vi "BRig_RT__Case_Exp__State_Cue.vi"(0 "input_dataCurrent":u16[](array[numeric]), 1 "input_dataTrial":u16[][](array[numeric]), 5 "input_arrTrig":bool[](array[boolean]), 6 "input_state":T1, 8 "I_lick":bool) -> (7 "output_l2_laserOn":bool, 9 "output_l2_laserEvent":bool, 10 "output_SelectionState":bool, 11 "output_l1_laserOn":bool, 12 "output_state":T1, 13 "output_l1_laserEvent":bool, 14 "output_dataCurrent":u16[](array[numeric]), 15 "output_dataTrial":u16[][](array[numeric]), 17 "output_CueLed":bool, 18 "output_Audio_L":bool, 19 "output_Audio_R":bool)   [LabVIEW 2014]
uses:
  myRIO_BRig_RT__Case_Exp_stateList.ctl
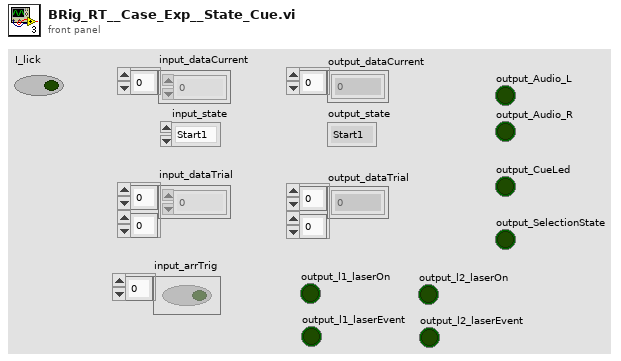
[diagram p1: front panel]
types:
  T1 = typedef "myRIO_BRig_RT__Case_Exp_stateList.ctl" = enum16{"Start1", "Start2", "Start3", "saveSettings1", "saveSettings2", "saveSettings3", "saveSettings4", "saveSettings_LC_ENL_l1", "saveSettings_LC_ENL_l2", "saveSettings_LC_Cue_l1", "saveSettings_LC_Cue_l2", "saveSettings6_LC_l1_Other", "SaveSettings6_LC_l2_Other", "setSettings_Audio", "setSettings_Laser", "initBlock_pre", "initBlock", "initBlock2", "initBlock_post", "initTrial_pre", "initTrial", "initTrial2", "initTrial3", "initTrial4", "initTrial_LC_ENL1", "initTrial_LC_Cue1", "initTrial_LC_Cue1_2", "initTrial_LC_Sel", "initTrial_post", "ENL1_pre", "ENL1", "ENL1_post", "ENL1Penalty_pre", "ENL1Penalty", "ENL2_pre", "ENL2", "ENL2Penalty_pre", "ENL2Penalty", "Cue1_pre", "Cue1", "Cue1_post", "Cue1Penalty_pre", "Cue1Penalty", "Cue2_pre", "Cue2", "Cue2Penalty_pre", "Cue2Penalty", "Selection_pre", "Selection", "Select_post", "SelectReward_pre", "SelectReward", "SelectRewardPost_pre", "SelectRewardPost", "SelectWrong_pre", "SelectWrong", "SelectWrong_post", "SelectTimeout_pre", "SelectTimeout", "SelectTimeout_post", "endTrial_pre", "endTrial1", "endTrial2", "endTrial3", "endTrial_post", "endBlock_pre", "endBlock", "endBlock_post", "endExp", "commConnect", "commUpload_pre", "commUpload_dataBlock", "commUpload_dataCurrent", "commUpload_dataExp", "commUpload_dataLC", "commUpload_dataTrial", "commUpload_post", "saveData_pre", "saveData_dataBlock", "saveData_dataCurrent", "saveData_dataExp", "saveData_dataLC", "saveData_dataTrial", "saveData_post", "empty_endBlock1", "empty_endBlock2", "empty_endTrial1", "empty_endTrial2", "empty_endTrial3", "empty_endTrial4", "empty_endTrial5", "dummyState", "dummyState_endBlock", "FreeReward_pre", "FreeReward", "FreeRewardPost_pre", "FreeRewardPost"}
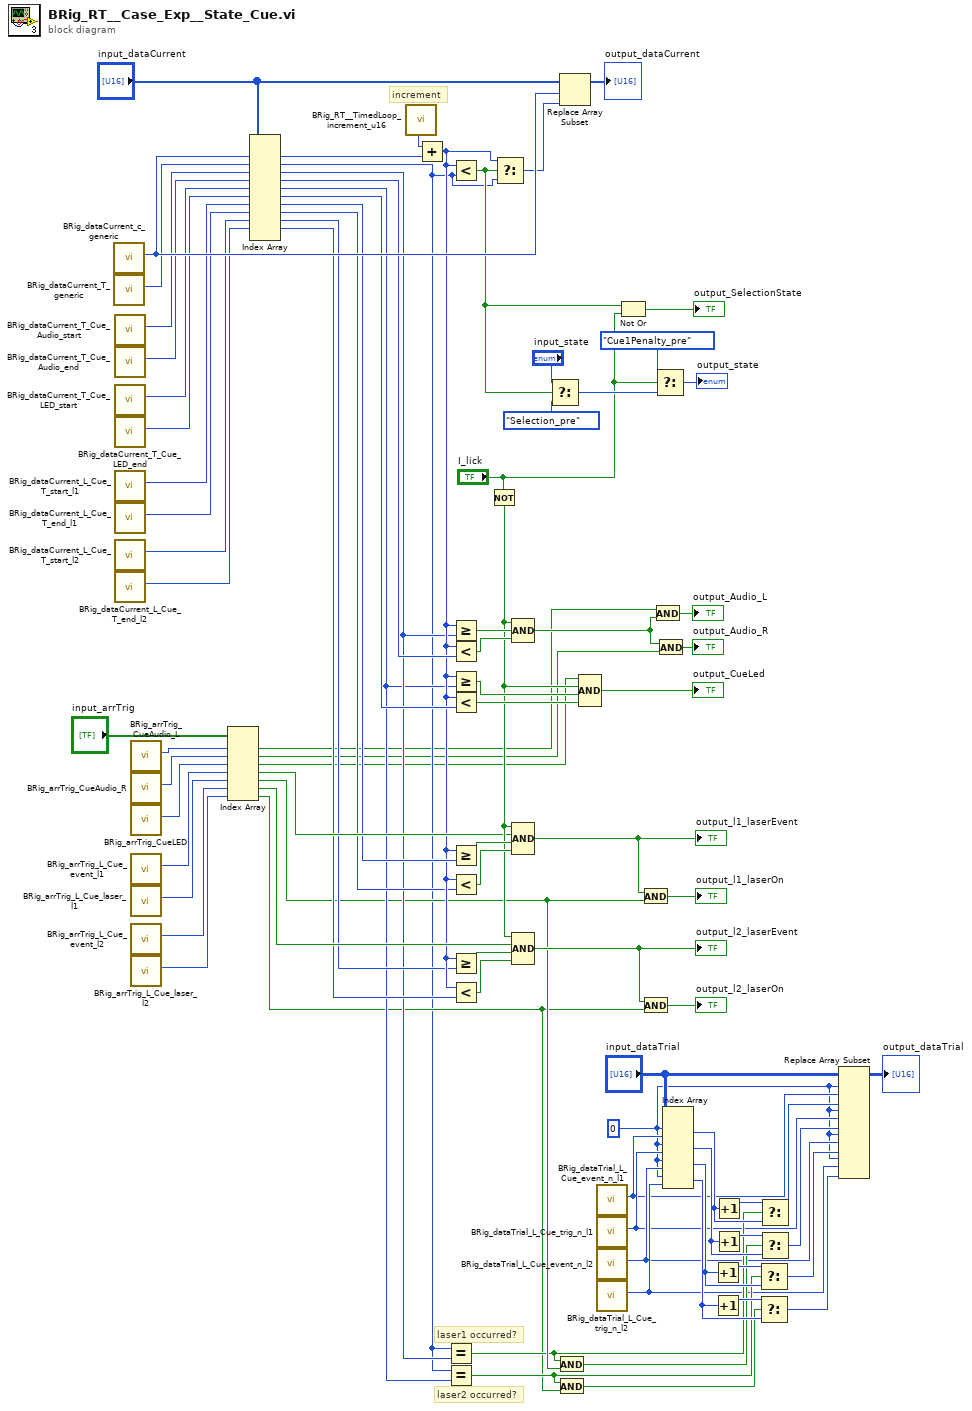
[diagram p0: block diagram]
diagram:
  w1 = 0
  # "laser2 occurred?"
  # "laser1 occurred?"
  # "increment"
  n1 = call "BRig_dataCurrent_c_generic.vi"() -> ("output_count_generic"=w66:i32)  [unwired: 11 in]
  n2 = call "BRig_dataCurrent_T_generic.vi"() -> ("output_T_generic"=w65:i32)  [unwired: 11 in]
  n3 = call "BRig_dataCurrent_T_Cue_Audio_start.vi"() -> ("output_T_Cue_Audio_start"=w64:i32)  [unwired: 11 in]
  n4 = call "BRig_dataCurrent_T_Cue_Audio_end.vi"() -> ("output_T_Cue_Audio_end"=w63:i32)  [unwired: 11 in]
  n5 = call "BRig_dataCurrent_T_Cue_LED_start.vi"() -> ("output_T_Cue_LED_start"=w61:i32)  [unwired: 11 in]
  n6 = call "BRig_dataCurrent_T_Cue_LED_end.vi"() -> ("output_T_Cue_LED_end"=w60:i32)  [unwired: 11 in]
  n7 = call "BRig_dataCurrent_L_Cue_T_start_l1.vi"() -> ("outputL_Cue_T_start_l1"=w46:i32)  [unwired: 11 in]
  n8 = call "BRig_dataCurrent_L_Cue_T_end_l1.vi"() -> ("output_L_Cue_T_end_l1"=w45:i32)  [unwired: 11 in]
  n9 = call "BRig_dataCurrent_L_Cue_T_start_l2.vi"() -> ("output_L_Cue_T_start_l2"=w44:i32)  [unwired: 11 in]
  n10 = call "BRig_dataCurrent_L_Cue_T_end_l2.vi"() -> ("output_L_Cue_T_end_l2"=w43:i32)  [unwired: 11 in]
  n11 = call "BRig_arrTrig_CueAudio_L.vi"() -> ("output_CueAudio_L"=w6:i32)  [unwired: 11 in]
  n12 = call "BRig_arrTrig_CueAudio_R.vi"() -> ("output_CueAudio_R"=w7:i32)  [unwired: 11 in]
  n13 = call "BRig_arrTrig_CueLED.vi"() -> ("output_CueLED"=w8:i32)  [unwired: 11 in]
  n14 = call "BRig_arrTrig_L_Cue_event_l1.vi"() -> ("output_L_Cue_event_l1"=w70:i32)  [unwired: 11 in]
  n15 = call "BRig_arrTrig_L_Cue_laser_l1.vi"() -> ("output_L_Cue_laser_l1"=w68:i32)  [unwired: 11 in]
  n16 = call "BRig_arrTrig_L_Cue_event_l2.vi"() -> ("output_L_Cue_event_l2"=w69:i32)  [unwired: 11 in]
  n17 = call "BRig_arrTrig_L_Cue_laser_l2.vi"() -> ("output_L_Cue_laser_l2"=w67:i32)  [unwired: 11 in]
  n18 = Index Array(array="input_arrTrig", index #1=w6, index #2=w7, index #3=w8, index #4=w70, index #5=w68, index #6=w69, index #7=w67) -> (element #1=w2:bool, element #2=w4:bool, element #3=w5:bool, element #4=w48:bool, element #5=w20:bool, element #6=w47:bool, element #7=w17:bool)
  n19 = Index Array(array="input_dataCurrent", index #1=w66, index #2=w65, index #3=w64, index #4=w63, index #5=w61, index #6=w60, index #7=w46, index #8=w45, index #9=w44, index #10=w43) -> (element #1=w62:u16, element #2=w10:u16, element #3=w22:u16, element #4=w54:u16, element #5=w21:u16, element #6=w53:u16, element #7=w42:u16, element #8=w39:u16, element #9=w38:u16, element #10=w37:u16)  [unwired: 1 in, 1 out]
  n20 = call "BRig_RT__TimedLoop_increment_u16.vi"() -> ("output_increment__u16"=w85:u16)  [unwired: 11 in]
  n21 = Add(x=w85, y=w62) -> (x+y=w41:u16)
  n22 = Equal?(x=w10, y=w22) -> (x = y?=w19:bool)
  n23 = Equal?(x=w10, y=w21) -> (x = y?=w18:bool)
  n24 = Less?(x=w41, y=w10) -> (x < y?=w40:bool)
  n25 = Greater Or Equal?(x=w41, y=w22) -> (x >= y?=w58:bool)
  n26 = Less?(x=w41, y=w54) -> (x < y?=w59:bool)
  n27 = Greater Or Equal?(x=w41, y=w21) -> (x >= y?=w56:bool)
  n28 = Less?(x=w41, y=w53) -> (x < y?=w55:bool)
  n29 = Greater Or Equal?(x=w41, y=w42) -> (x >= y?=w83:bool)
  n30 = Less?(x=w41, y=w39) -> (x < y?=w84:bool)
  n31 = Greater Or Equal?(x=w41, y=w38) -> (x >= y?=w75:bool)
  n32 = Less?(x=w41, y=w37) -> (x < y?=w74:bool)
  n33 = Not(x="I_lick") -> (.not. x?=w49:bool)
  n34 = Select(t=w41, s=w40, f=w10) -> (s? t:f=w57:u16)
  n35 = Compound Arithmetic op=AND(w49, w58, w59) -> (w3:bool)
  n36 = Compound Arithmetic op=AND(w49, w48, w83, w84) -> (w77:bool)
  "output_l1_laserEvent" <- w77
  n37 = Compound Arithmetic op=AND(w49, w47, w75, w74) -> (w73:bool)
  "output_l2_laserEvent" <- w73
  n38 = Select(t="input_state", s=w40, f=myRIO_BRig_RT__Case_Exp_stateList."Selection_pre" ("Enum")) -> (s? t:f=w86:T1)
  n39 = And(x=w19, y=w20) -> (x .and. y?=w16:bool)
  n40 = And(x=w18, y=w17) -> (x .and. y?=w15:bool)
  n41 = Replace Array Subset(array="input_dataCurrent", new element=w57, index=w66) -> (→"output_dataCurrent":u16[])
  n42 = Compound Arithmetic op=AND(w5, w49, w56, w55) -> (→"output_CueLed":bool)
  n43 = call "BRig_dataTrial_L_Cue_event_n_l1.vi"() -> ("output_L_Cue_event_n_l1"=w11:i32)  [unwired: 11 in]
  n44 = call "BRig_dataTrial_L_Cue_trig_n_l1.vi"() -> ("output_L_Cue_trig_n_l1"=w12:i32)  [unwired: 11 in]
  n45 = call "BRig_dataTrial_L_Cue_event_n_l2.vi"() -> ("output_L_Cue_event_n_l2"=w13:i32)  [unwired: 11 in]
  n46 = call "BRig_dataTrial_L_Cue_trig_n_l2.vi"() -> ("output_L_Cue_trig_n_l2"=w14:i32)  [unwired: 11 in]
  n47 = Not Or(1:"I_lick", 2:w40) -> (0:→"output_SelectionState":bool)
  n48 = And(x=w77, y=w20) -> (x .and. y?=→"output_l1_laserOn":bool)
  n49 = And(x=w73, y=w17) -> (x .and. y?=→"output_l2_laserOn":bool)
  n50 = And(x=w2, y=w3) -> (x .and. y?=→"output_Audio_L":bool)
  n51 = Select(t=myRIO_BRig_RT__Case_Exp_stateList."Cue1Penalty_pre" ("Enum"), s="I_lick", f=w86) -> (s? t:f=→"output_state":T1)
  n52 = And(x=w3, y=w4) -> (x .and. y?=→"output_Audio_R":bool)
  n53 = Index Array(array="input_dataTrial", index (row) #1=w1, index (col) #1=w11, index (row) #2=w1, index (col) #2=w12, index (row) #3=w1, index (col) #3=w13, index (row) #4=w1, index (col) #4=w14) -> (element #1=w34:u16, element #2=w30:u16, element #3=w29:u16, element #4=w28:u16)
  n54 = Increment(x=w29) -> (x+1=w32:u16)
  n55 = Increment(x=w28) -> (x+1=w31:u16)
  n56 = Increment(x=w34) -> (x+1=w35:u16)
  n57 = Increment(x=w30) -> (x+1=w33:u16)
  n58 = Select(t=w32, s=w18, f=w29) -> (s? t:f=w25:u16)
  n59 = Select(t=w31, s=w15, f=w28) -> (s? t:f=w24:u16)
  n60 = Select(t=w35, s=w19, f=w34) -> (s? t:f=w27:u16)
  n61 = Select(t=w33, s=w16, f=w30) -> (s? t:f=w26:u16)
  n62 = Replace Array Subset(array="input_dataTrial", new element #1=w27, index (row) #1=w1, index (col) #1=w11, new element #2=w26, index (row) #2=w1, index (col) #2=w12, new element #3=w25, index (row) #3=w1, index (col) #3=w13, new element #4=w24, index (row) #4=w1, index (col) #4=w14) -> (→"output_dataTrial":u16[][])
